vi "FTW-Endpoint-Multipart-Receive.vi"(0 "FTW Endpoint":refnum<class "FTW-Endpoint-HTTP.lvclass">, 5 "Timeout":i32 format="%dmsec", 11 "error in":errorcluster) -> (4 "FTW Endpoint out":refnum<class "FTW-Endpoint-HTTP.lvclass">, 6 "Message Received":T1, 8 "Timed out?":bool, 15 "error out":errorcluster)   [LabVIEW 2015, in "FTW-Endpoint-HTTP.lvclass"]
uses:
  FTW-Endpoint-HTTP.lvclass
  Payload/FTW-MessagePayload.ctl
panel:
  # "Inputs"
  # "Outputs"
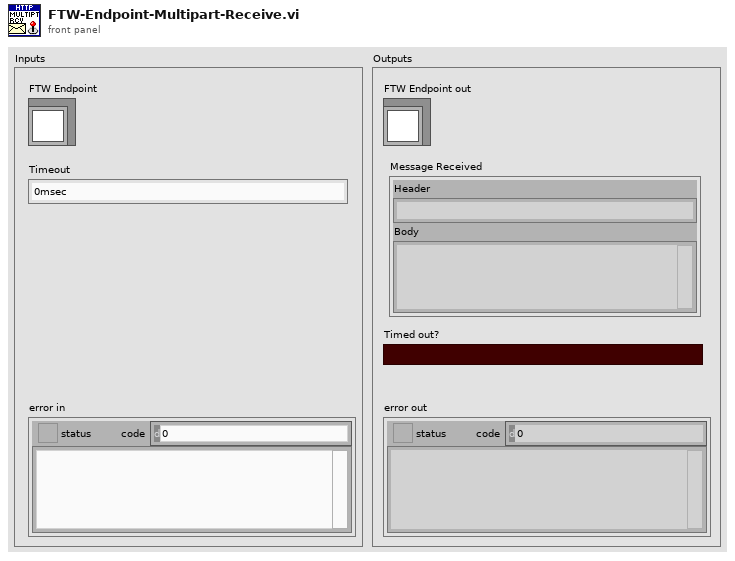
[diagram p1: front panel]
types:
  T1 = typedef "FTW-MessagePayload.ctl" = cluster{"Header":string, "Body":string, "FTW: Sender Identity":string, "FTW: Reply Address":string, "FTW: Reply Error":errorcluster}
  T2 = enum16{"Standard", "Buffered", "CRLF", "Immediate"}
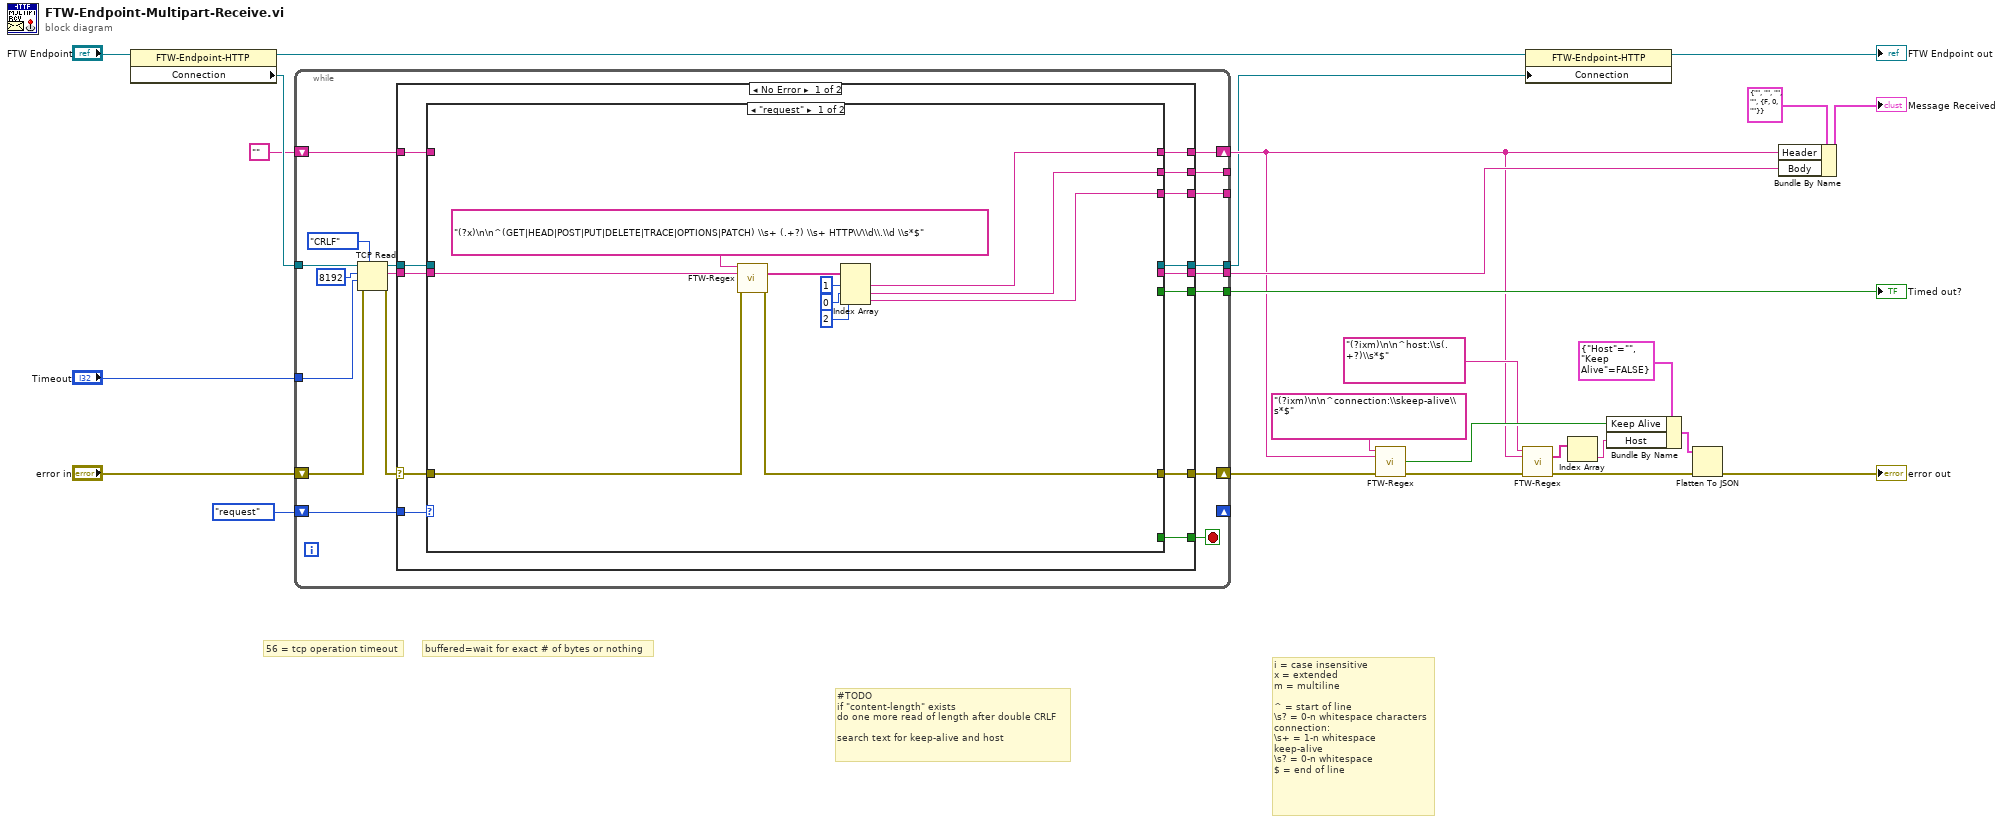
[diagram p0: block diagram]
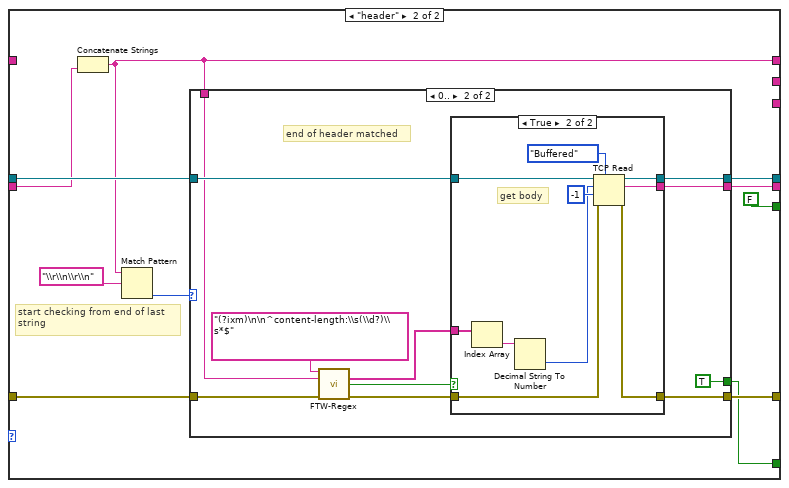
[diagram p2: hidden frame]
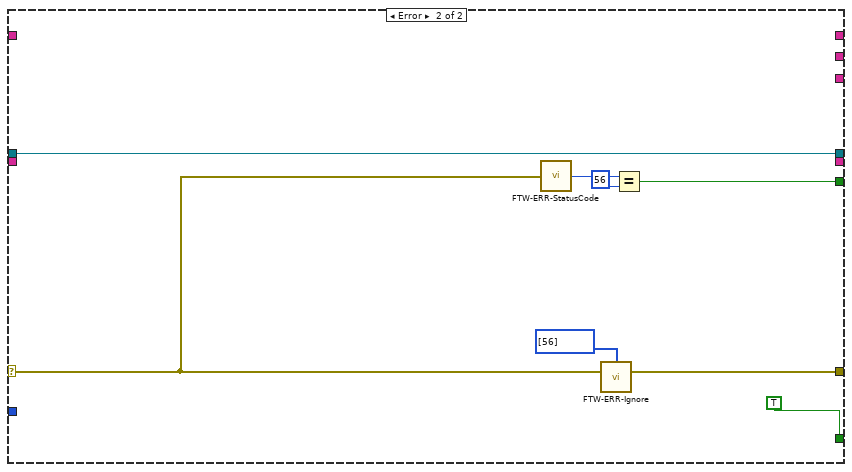
[diagram p5: hidden frame]
diagram:
  # "#TODO\nif \"content-length\" exists\ndo one more read of length after double CRLF\n\nsearch text for keep-alive and host"
  # "i = case insensitive\nx = extended\nm = multiline\n\n^ = start of line\n\\s? = 0-n whitespace characters\nconnection:\n\\s+ = 1-n whitespace\nkeep-alive\n\\s? = 0-n whitespace\n$ = end of line"
  # "buffered=wait for exact # of bytes or nothing"
  # "56 = tcp operation timeout"
  n1 = property class="FTW-Endpoint-HTTP"(reference="FTW Endpoint") -> (reference out=w6:refnum<class "FTW-Endpoint-HTTP.lvclass">, "Connection"=w5:refnum<k5>)  [unwired: 1 in, 1 out]
  n2 = while {
    tunnel: w5 -> [w39]
    tunnel: [w38] -> w7
    tunnel: [w36] -> w20
    shift-right: [w37] -> w19
    shift-left: "error in" -> [w34]
    tunnel: [w30] -> w13
    tunnel: "Timeout" -> [w33]
    shift-right: _ -> [_]
    shift-left: enum16{"request", "header", "body"}."request" -> [w29]
    shift-right: [w32] -> w10
    shift-left: "" ("empty string") -> [w28]
    tunnel: [w27] -> _
    tunnel: [w26] -> _
    stop <- w31 stop-if-true
    n3 = TCP Read(connection ID=w39, bytes to read=8192, error in (no error)=w34, 7:T2."CRLF" ("mode (standard)"), 9:w33) -> (connection ID out=w41:refnum<k5>, data out=w35:string, error out=w42:errorcluster)
    n4 = case shown="No Error" w42 {
      selector: w42 -> [w52 w109]
      tunnel: w41 -> [w56 w107]
      tunnel: [w54 w107] -> w38
      tunnel: [w51 w108] -> w37
      tunnel: [w50 w110] -> w36
      tunnel: w35 -> [w55 _]
      tunnel: [w48 w106] -> w32
      tunnel: [w49 TRUE] -> w31
      tunnel: [w53 _] -> w30
      tunnel: w29 -> [w47 _]
      tunnel: w28 -> [w46 _]
      tunnel: [w45 _] -> w27
      tunnel: [w44 _] -> w26
      frame No Error {
        n5 = case shown="\"request\"" w47 {
          tunnel: w56 -> [_ w79]
          tunnel: w55 -> [w66 w78]
          tunnel: [_ w76] -> w54
          tunnel: [_ w75] -> w53
          tunnel: w52 -> [w65 w74]
          tunnel: [w64 w73] -> w51
          tunnel: [_ FALSE] -> w50
          tunnel: [_ w69] -> w49
          tunnel: [w59 w68] -> w48
          tunnel: w46 -> [_ _]
          tunnel: [w58 _] -> w45
          tunnel: [w57 _] -> w44
          frame "request" {
            n6 = call "FTW-Regex.vi"("Regular Expression"="(?x)\n\n^(GET|HEAD|POST|PUT|DELETE|TRACE|OPTIONS|PATCH) \\s+ (.+?) \\s+ HTTP\\/\\d\\.\\d \\s*$", "Input String"=w66, "error in"=w65) -> ("Submatches"=w63:string[], "error out"=w64:errorcluster)  [unwired: 8 in, 3 out]
            n7 = Index Array(array=w63, index #1=1 ("index"), index #2=0 ("index"), index #3=2 ("index")) -> (element #1=w59:string, element #2=w58:string, element #3=w57:string)
          }
          frame "header" {
            # "start checking from end of last\nstring"
            n8 = Concatenate Strings(w78) -> (w68:string, w71:string)
            n9 = Match Pattern(string=w68, regular expression="\\r\\n\\r\\n") -> (offset past match=w70:i32)  [unwired: 1 in, 3 out]
            n10 = case shown="0.." w70 {
              tunnel: w79 -> [w81 w92]
              tunnel: [w81 w91] -> w76
              tunnel: [_ w90] -> w75
              tunnel: w74 -> [w80 w88]
              tunnel: [w80 w86] -> w73
              tunnel: [_ TRUE] -> w69
              tunnel: w68 -> [_ w82]
              frame ..-1 {
                # "end of header not found, keep looking"
              }
              frame 0.. {
                # "end of header matched"
                n11 = call "FTW-Regex.vi"("Regular Expression"="(?ixm)\n\n^content-length:\\s(\\d?)\\s*$", "Input String"=w82, "error in"=w88) -> ("Submatches"=w84:string[], "Match Found?"=w83:bool, "error out"=w87:errorcluster)  [unwired: 8 in, 2 out]
                n12 = case shown="True" w83 {
                  tunnel: w92 -> [w94 w104]
                  tunnel: [w94 w103] -> w91
                  tunnel: [_ w102] -> w90
                  tunnel: w87 -> [w93 w101]
                  tunnel: [w93 w100] -> w86
                  tunnel: w84 -> [_ w97]
                  frame False {
                    # "content length not found"
                  }
                  frame True {
                    # "get body"
                    n13 = Index Array(array=w97) -> (element=w96:string)  [unwired: 1 in]
                    n14 = Decimal String To Number(string=w96) -> (number=w95:i32)  [unwired: 2 in, 1 out]
                    n15 = TCP Read(connection ID=w104, bytes to read=w95, error in (no error)=w101, 7:T2."Buffered" ("mode (standard)"), 9:-1 ("timeout ms (25000)")) -> (connection ID out=w103:refnum<k5>, data out=w102:string, error out=w100:errorcluster)
                  }
                }
              }
            }
          }
        }
      }
      frame Error {
        n16 = call "FTW-ERR-StatusCode.vi"("error to check"=w109) -> ("Code"=w113:i32)
        n17 = call "FTW-ERR-Ignore.vi"("Codes to filter"=i32[] [56], "error to filter"=w109) -> ("filtered error"=w108:errorcluster)  [unwired: 13 in]
        n18 = Equal?(x=w113, y=56 ("x")) -> (x = y?=w110:bool)
      }
    }
  }
  "Timed out?" <- w20
  n19 = call "FTW-Regex.vi"("Regular Expression"="(?ixm)\n\n^connection:\\skeep-alive\\s*$", "Input String"=w10, "error in"=w19) -> ("Match Found?"=w14:bool, "error out"=w16:errorcluster)  [unwired: 8 in, 3 out]
  n20 = call "FTW-Regex.vi"("Regular Expression"="(?ixm)\n\n^host:\\s(.+?)\\s*$", "Input String"=w10, "error in"=w16) -> ("Submatches"=w9:string[], "error out"=w12:errorcluster)  [unwired: 8 in, 3 out]
  n21 = property class="FTW-Endpoint-HTTP"(reference=w6, "Connection"=w7) -> (reference out=→"FTW Endpoint out":refnum<class "FTW-Endpoint-HTTP.lvclass">)  [unwired: 1 in, 1 out]
  n22 = Index Array(array=w9) -> (element=w8:string)  [unwired: 1 in]
  n23 = Bundle By Name(cluster=cluster{"Host":string, "Keep Alive":bool} {"Host"="", "Keep Alive"=FALSE}, "Keep Alive"=w14, "Host"=w8) -> (w17:cluster{"Host":string, "Keep Alive":bool})
  n24 = Flatten To JSON(anything=w17, error in (no error)=w12) -> (11:→"error out":errorcluster)  [unwired: 1 in, 1 out]
  n25 = Bundle By Name(cluster=T1 {"Header"="", "Body"="", "FTW: Sender Identity"="", "FTW: Reply Address"="", "FTW: Reply Error"={"status"=FALSE, "code"=0, "source"=""}} ("Message Received"), "Header"=w10, "Body"=w13) -> (→"Message Received":T1)
